vi "Keithley 6514 Filter Config.vi"(0 "Resource In":refnum<visa-resource-name>, 1 "Check For SCPI Errors? (T)":bool=TRUE, 5 "digital filter type (None:0)":u16(ring) items=["None (filter off)", "Averaging", "Advanced"], 7 "filter type control (Moving:0)":u16(ring) items=["Moving", "Repeat"], 9 "dig. filter count":i16=10 min=2 max=100 step=1, 11 "error in (no error)":T1, 12 "noise tolerance (%)":dbl min=0.0 max=105.0 step=0.01 format="%.3f", 13 "Median":u16(ring) items=["Off", "On"], 14 "Median Rank":i16=1 min=1 max=5 step=1) -> (4 "Resource Out (dupl)":refnum<visa-resource-name>, 15 "error out":T1)   [LabVIEW 2009, in "Keithley 6514 LV 2009.lvlib"]
doc: "This VI is used to configure the settings for the Averaging Filters. Refer to the Instrument manual for complete details on the filters.\n\ndigital filter type:\n0 = none (filter off)\n1 = Averaging filter on\n2 = Averaging and Advanced Filters on\n\nfilter type control:\n0 = Moving\n1 = Repeat\n\ndigital filter count:\n2 to 100\n\nnoise tolerance (%):\n0 to 105\n\nMedian:\n0 = Off\n1 = On\n\nMedian Rank:\n1 to 5"
uses:
  Keithley 6514 LV 2009.lvlib
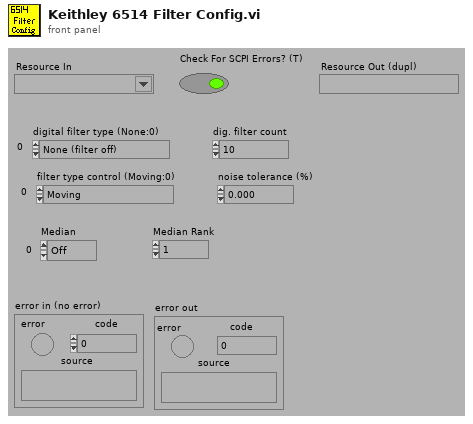
[diagram p1: front panel]
types:
  T1 = cluster{"error":bool, "code":i32, "source":string}
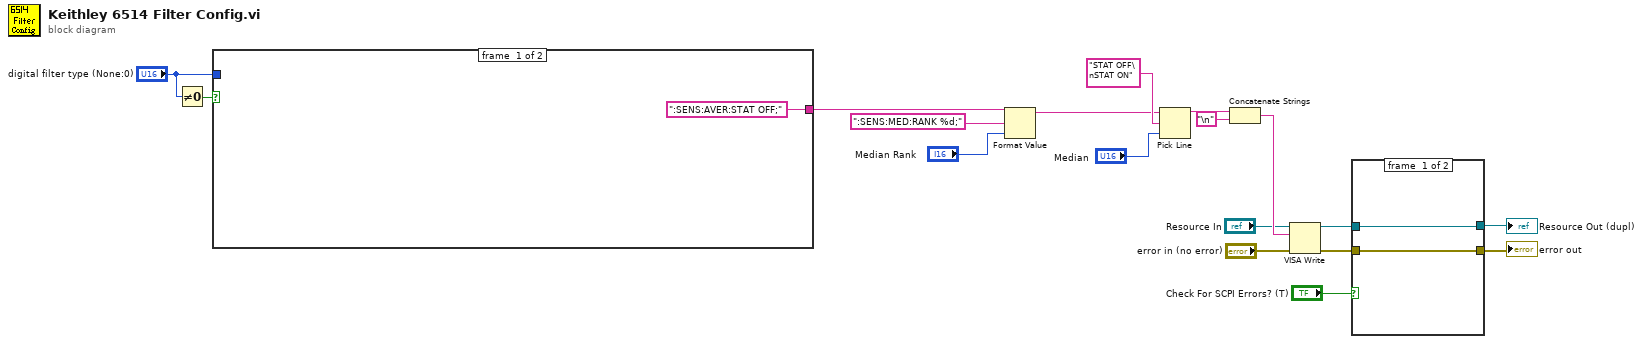
[diagram p0: block diagram]
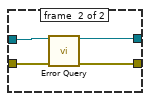
[diagram p2: hidden frame]
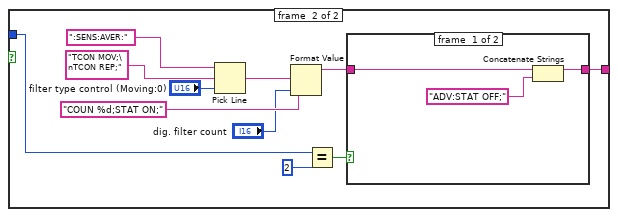
[diagram p3: hidden frame]
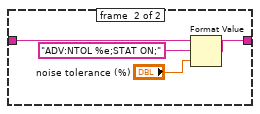
[diagram p4: hidden frame]
diagram:
  n1 = Not Equal To 0?(x="digital filter type (None:0)") -> (x != 0?=w14:bool)
  n2 = case shown="True" w14 {
    tunnel: "digital filter type (None:0)" -> [_ w23]
    tunnel: [":SENS:AVER:STAT OFF;" w20] -> w12
    frame #0 {
    }
    frame #1 {
      n3 = Pick Line(string ("")=":SENS:AVER:", multi-line string="TCON MOV;\nTCON REP;", line index="filter type control (Moving:0)") -> (output string=w26:string)
      n4 = Format Value(string ("")=w26, format string="COUN %d;STAT ON;", value (0)="dig. filter count") -> (output string=w21:string)
      n5 = Equal?(x=w23, y=u16 2) -> (x = y?=w22:bool)
      n6 = case shown="False" w22 {
        tunnel: w21 -> [w32 w36]
        tunnel: [w31 w34] -> w20
        frame #0 {
          n7 = Concatenate Strings(w32, "ADV:STAT OFF;") -> (w31:string)
        }
        frame #1 {
          n8 = Format Value(string ("")=w36, format string="ADV:NTOL %e;STAT ON;", value (0)="noise tolerance (%)") -> (output string=w34:string)
        }
      }
    }
  }
  n9 = Format Value(string ("")=w12, format string=":SENS:MED:RANK %d;", value (0)="Median Rank") -> (output string=w11:string)
  n10 = Pick Line(string ("")=w11, multi-line string="STAT OFF\nSTAT ON", line index="Median") -> (output string=w1:string)
  n11 = Concatenate Strings(w1, "\n") -> (w9:string)
  n12 = VISA Write(VISA resource name="Resource In", write buffer=w9, error in (no error)="error in (no error)") -> (VISA resource name out=w5:refnum<visa-resource-name>, error out=w4:errorcluster)  [unwired: 1 out]
  n13 = case shown="False" "Check For SCPI Errors? (T)" {
    tunnel: w5 -> [w39 w43]
    tunnel: w4 -> [w38 w42]
    tunnel: [w39 w41] -> w3
    tunnel: [w38 w40] -> w2
    frame #0 {
    }
    frame #1 {
      n14 = call "Error Query.vi"("VISA Resource In"=w43, "error in (no error)"=w42) -> ("VISA Resource Out (dupl)"=w41:refnum<visa-resource-name>, "error out"=w40:errorcluster)  [unwired: 10 in, 2 out]
    }
  }
  "error out" <- w2
  "Resource Out (dupl)" <- w3
